vi "Log Result.vi"(8 "error in (no error)":errorcluster, 10 "Result":refnum<class "Acquired Result.lvclass">, 11 "File in":refnum<class "File.lvclass">) -> (0 "error out":errorcluster, 3 "File out":refnum<class "File.lvclass">)   [LabVIEW 2019, in "File.lvclass"]
uses:
  File.lvclass
  Instruments/Results/Acquired Result/Acquired Result.lvclass
  File.lvclass/File.ctl
  Read tdms stream.vi
  Read Is open.vi
  Read Timestamp data points.vi
  Write tdms stream.vi
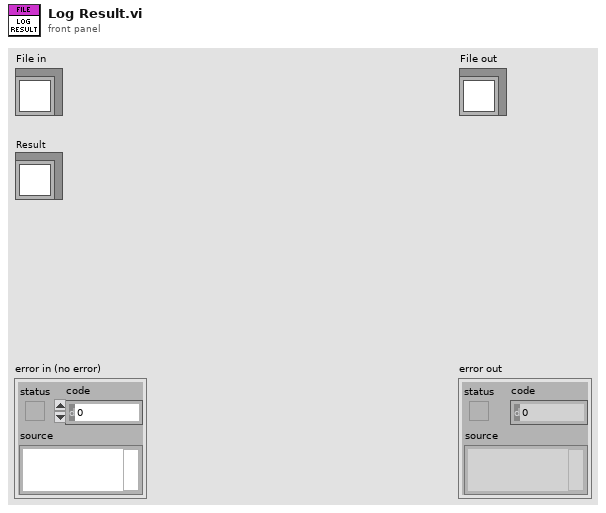
[diagram p1: front panel]
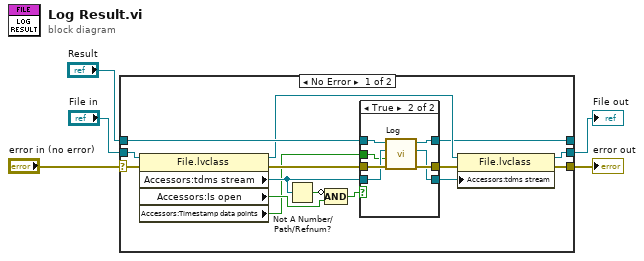
[diagram p0: block diagram]
diagram:
  n1 = case shown="No Error" "error in (no error)" {
    selector: "error in (no error)" -> [w17 w33]
    tunnel: [w16 w33] -> w2
    tunnel: [w12 w32] -> w3
    tunnel: "File in" -> [w13 w32]
    tunnel: "Result" -> [w15 w31]
    tunnel: [w11 w31] -> _
    frame No Error {
      n2 = property class="File.lvclass"(reference=w13, error in=w17) -> (reference out=w14:refnum<class "File.lvclass">, error out=w19:errorcluster, "Accessors:tdms stream"=w10:refnum<k34>, "Accessors:Is open"=w7:bool, "Accessors:Timestamp data points"=w6:bool)
      n3 = Not A Number/Path/Refnum?(number/path/refnum=w10) -> (NaN/Path/Refnum?=w9:bool)
      n4 = Compound Arithmetic op=AND(invert w9, w7) -> (w8:bool)
      n5 = case shown="True" w8 {
        tunnel: [w23 w30] -> w20
        tunnel: w19 -> [w23 w29]
        tunnel: [w21 w28] -> w18
        tunnel: w10 -> [w21 w27]
        tunnel: w15 -> [w22 w26]
        tunnel: [w22 w25] -> w11
        tunnel: w6 -> [_ w24]
        frame False {
        }
        frame True {
          n6 = call-dynamic "Log.vi"("error in (no error)"=w29, "Timestamp data points"=w24, "tdms file"=w27, "Acquired Result in"=w26) -> ("error out"=w30:errorcluster, "tdms file out"=w28:refnum<k34>, "Acquired Result out"=w25:refnum<class "Acquired Result.lvclass">)  [unwired: 5 in]
        }
      }
      n7 = property class="File.lvclass"(reference=w14, error in=w20, "Accessors:tdms stream"=w18) -> (reference out=w12:refnum<class "File.lvclass">, error out=w16:errorcluster)
    }
    frame Error {
    }
  }
  "error out" <- w2
  "File out" <- w3
